vi "CAN 6 TalonSRX Motor Set PIDF with Gearing.vi"(9 "PIDF gains Low Gear":T1, 10 "PIDF gains High Gear":T1, 11 "TalonSRX6MotorRef":T2) -> (3 "TalonSRX6MotorRef":T2)   [LabVIEW 2017]
uses:
  TalonSRX6Motor.ctl
  <vilib>/Rock Robotics/WPI/MotorControl/WPI_MotorControlDeviceRef.ctl
  <vilib>/Rock Robotics/WPI/MotorControl/WPI_MotorControlType.ctl
  <vilib>/Rock Robotics/SystemInterfaces/DIO/FPGA_DIOPWMChannel.ctl
  <vilib>/Rock Robotics/WPI/PWM/WPI_PWMDeadband.ctl
  <vilib>/Rock Robotics/SystemInterfaces/DIO/FPGA_DIOChannel.ctl
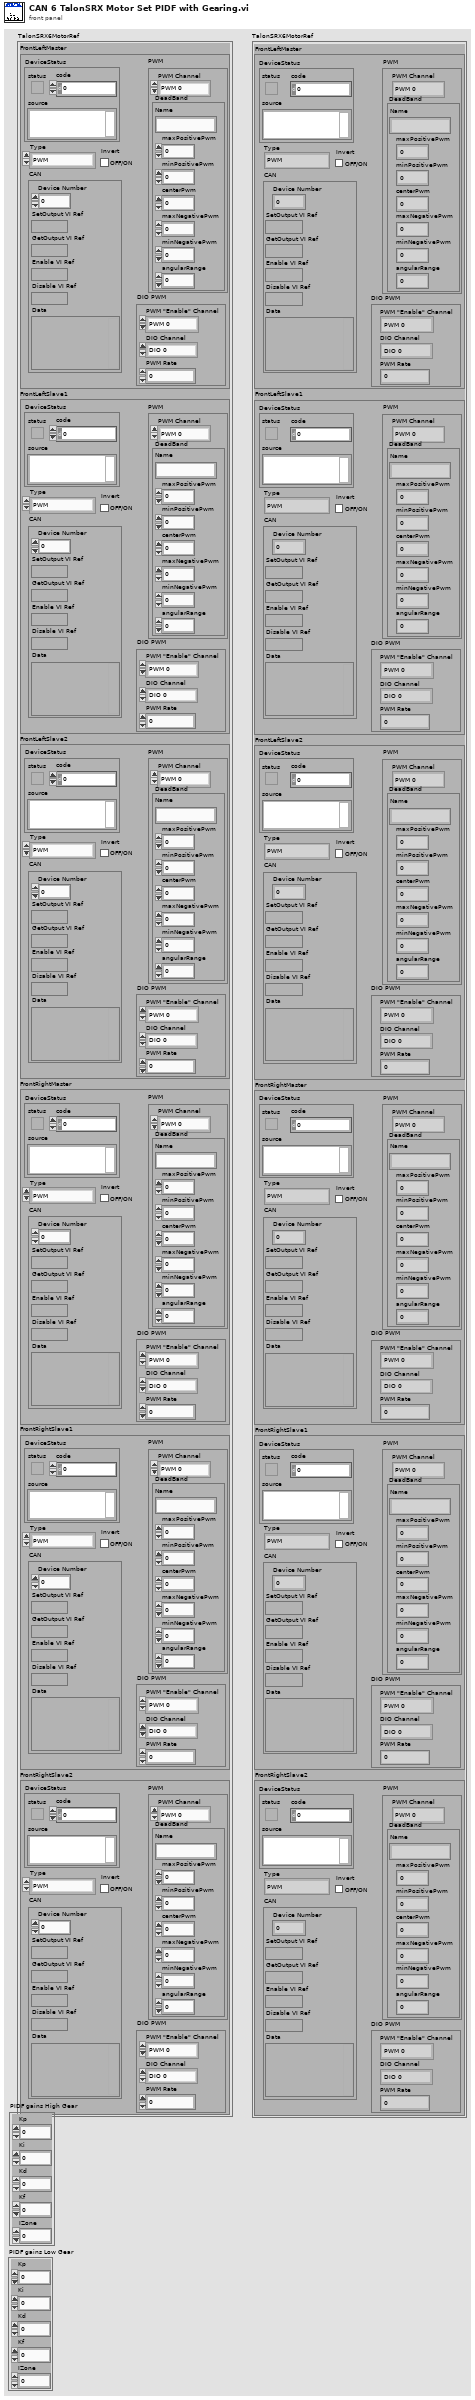
[diagram p1: front panel]
types:
  T1 = cluster{"Kp":dbl, "Ki":dbl, "Kd":dbl, "Kf":dbl, "IZone":dbl}
  T2 = typedef "TalonSRX6Motor.ctl" = cluster{"FrontLeftMaster":T3, "FrontLeftSlave1":T3, "FrontLeftSlave2":T3, "FrontRightMaster":T3, "FrontRightSlave1":T3, "FrontRightSlave2":T3}
  T3 = typedef "WPI_MotorControlDeviceRef.ctl" = cluster{"DeviceStatus":errorcluster, "Type":T4, "PWM":cluster{"PWM Channel":T5, "DeadBand":T6}, "CAN":cluster{"Device Number":u8, "SetOutput VI Ref":variant, "GetOutput VI Ref":variant, "Enable VI Ref":variant, "Disable VI Ref":variant, "Data":variant}, "Invert":bool, "DIO PWM":cluster{"PWM \"Enable\" Channel":T5, "DIOChannel":T7, "PWM Rate":dbl}}
  T4 = typedef "WPI_MotorControlType.ctl" = enum16{"PWM", "CAN", "DIO PWM"}
  T5 = typedef "FPGA_DIOPWMChannel.ctl" = enum8{"PWM 0", "PWM 1", "PWM 2", "PWM 3", "PWM 4", "PWM 5", "PWM 6", "PWM 7", "PWM 8", "PWM 9", "PWM MXP 0", "PWM MXP 1", "PWM MXP 2", "PWM MXP 3", "PWM MXP 4", "PWM MXP 5", "PWM MXP 6", "PWM MXP 7", "PWM MXP 8", "PWM MXP 9", "Invalid"}
  T6 = typedef "WPI_PWMDeadband.ctl" = cluster{"Name":string, "maxPositivePwm":i32, "minPositivePwm":i32, "centerPwm":i32, "maxNegativePwm":i32, "minNegativePwm":i32, "angularRange":u16}
  T7 = typedef "FPGA_DIOChannel.ctl" = enum8{"DIO 0", "DIO 1", "DIO 2", "DIO 3", "DIO 4", "DIO 5", "DIO 6", "DIO 7", "DIO 8", "DIO 9", "DIO MXP 0", "DIO MXP 1", "DIO MXP 2", "DIO MXP 3", "DIO MXP 4", "DIO MXP 5", "DIO MXP 6", "DIO MXP 7", "DIO MXP 8", "DIO MXP 9", "DIO MXP 10", "DIO MXP 11", "DIO MXP 12", "DIO MXP 13", "DIO MXP 14", "DIO MXP 15", "SPI Port CS1", "SPI Port CS2", "SPI Port CS3", "SPI Port MISO", "SPI Port MOSI", "Invalid"}
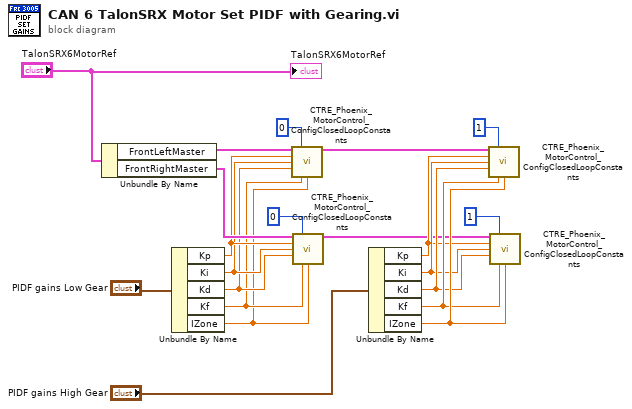
[diagram p0: block diagram]
diagram:
  n1 = Unbundle By Name("TalonSRX6MotorRef") -> ("FrontLeftMaster"=w20:T3, "FrontRightMaster"=w21:T3)
  n2 = Unbundle By Name("PIDF gains Low Gear") -> ("Kp"=w16:dbl, "Ki"=w15:dbl, "Kd"=w14:dbl, "Kf"=w13:dbl, "IZone"=w12:dbl)
  n3 = call <vilib>:"CTRE_Phoenix_MotorControl_ConfigClosedLoopConstants.vi"("PhoenixMotorControlDevRef"=w20, "slotIdx"=0, "P"=w16, "I"=w15, "D"=w14, "F"=w13, "I Zone"=w12) -> ("PhoenixMotorControlDevRef"=w3:T3)  [unwired: 7 in, 1 out]
  n4 = call <vilib>:"CTRE_Phoenix_MotorControl_ConfigClosedLoopConstants.vi"("PhoenixMotorControlDevRef"=w21, "slotIdx"=0, "P"=w16, "I"=w15, "D"=w14, "F"=w13, "I Zone"=w12) -> ("PhoenixMotorControlDevRef"=w4:T3)  [unwired: 7 in, 1 out]
  n5 = Unbundle By Name("PIDF gains High Gear") -> ("Kp"=w6:dbl, "Ki"=w7:dbl, "Kd"=w8:dbl, "Kf"=w9:dbl, "IZone"=w10:dbl)
  n6 = call <vilib>:"CTRE_Phoenix_MotorControl_ConfigClosedLoopConstants.vi"("PhoenixMotorControlDevRef"=w3, "slotIdx"=1, "P"=w6, "I"=w7, "D"=w8, "F"=w9, "I Zone"=w10) -> ()  [unwired: 7 in, 2 out]
  n7 = call <vilib>:"CTRE_Phoenix_MotorControl_ConfigClosedLoopConstants.vi"("PhoenixMotorControlDevRef"=w4, "slotIdx"=1, "P"=w6, "I"=w7, "D"=w8, "F"=w9, "I Zone"=w10) -> ()  [unwired: 7 in, 2 out]
  "TalonSRX6MotorRef" <- "TalonSRX6MotorRef"
